vi "Teleop.vi"(10 "Match Info":T1={"Autonomous Elapsed Seconds"=0.0, "TeleOp Elapsed Seconds"=0.0, "Disabled Elapsed Seconds"=0.0, "Visited Autonomous"=FALSE, "Visited TeleOp"=FALSE, "Visited Disabled"=FALSE, "Autonomous Settings"={"Autonomous Style"=enum."Independent", "VI Refnum"=refnum}}, 11 "Call Context":T2) -> ()   [LabVIEW 2012]
doc: "This VI is called for each TeleOp packet received from the DS where the robot is not disabled. It is often used to read from the joysticks and update I/O or to update setpoints for timed control loops. It should complete and return within 20 milliseconds or it may miss DS packets."
uses:
  <vilib>/Rock Robotics/WPI/DriverStation/WPI_DriverStationDerivedRobotMode.ctl
  <vilib>/Rock Robotics/WPI/DriverStation/WPI_DriverStationMatch Info.ctl
  Desktop/Code 2013/ king-kong-2230-2013/Robot Global Data.vi
  <vilib>/Rock Robotics/WPI/RobotDrive/WPI_RobotDriveGetSetRefNum.vi
panel:
  in  "Telescopic Toghether?":bool
  in  "Cannons Toghether?":bool
  in  "Cananot Toghether?":bool
  in  "2  Cananot (Climb)":dbl(slide) scale=-1.0..1.0
  in  "2  Telescopic(Climb)":dbl(slide) scale=-1.0..1.0
  in  "2 Cannons":dbl(slide) scale=-1.0..1.0
  in  "Flipper Servos":i32(knob) scale=0.0..170.0
  in  "Feeder Servos":i32(knob) scale=0.0..160.0
  in  "Climb Telescopic Right":dbl(slide) scale=-1.0..1.0
  in  "Climb Telescopic Left":dbl(slide) scale=-1.0..1.0
  in  "Transfer":dbl(slide) scale=-1.0..1.0
  in  "Canenet Left":dbl(slide) scale=-1.0..1.0
  in  "Canenet Right":dbl(slide) scale=-1.0..1.0
  in  "Conveyer Belt":dbl(slide) scale=-1.0..1.0
  in  "zAvit":dbl(slide) scale=-1.0..1.0
  in  "First Cannon":dbl(slide) scale=-1.0..1.0
  in  "Second Cannon":dbl(slide) scale=-1.0..1.0
  in  "Y axis value":dbl(slide) scale=-1.0..1.0
  in  "X axis value":dbl(slide) scale=-1.0..1.0
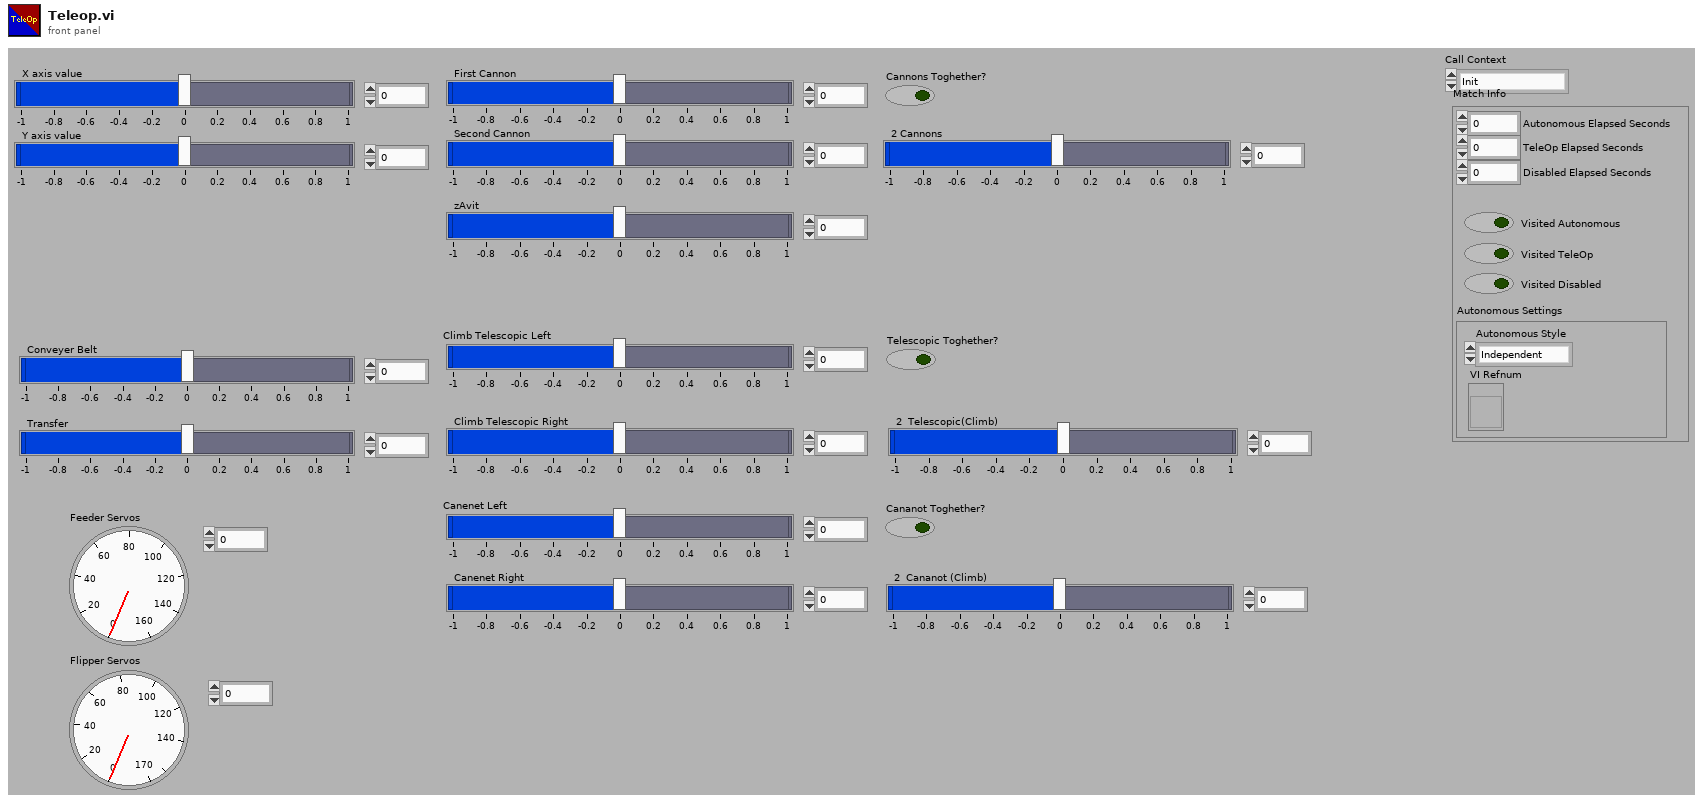
[diagram p1: front panel]
types:
  T1 = typedef "WPI_DriverStationMatch Info.ctl" = cluster{"Autonomous Elapsed Seconds":dbl, "TeleOp Elapsed Seconds":dbl, "Disabled Elapsed Seconds":dbl, "Visited Autonomous":bool, "Visited TeleOp":bool, "Visited Disabled":bool, "Autonomous Settings":cluster{"Autonomous Style":enum16{"Iterative", "Independent"}, "VI Refnum":refnum<vi>}}
  T2 = typedef "WPI_DriverStationDerivedRobotMode.ctl" = enum16{"Init", "Execute", "Stop"}
  T3 = typedef "WPI_MotorControlDeviceRef.ctl" = cluster{"DeviceStatus":errorcluster, "Type":enum16{"PWM", "CAN"}, "PWM":cluster{"Digital Module":T4, "PWM Channel":T5, "DeadBand":T6}, "CAN":cluster{"Device Number":u8, "Control Mode":T7, "Semaphore":T8, "Max Vout":dbl}, "Invert":bool, "TransformRef":T9, "InvTransformRef":T9}
  T4 = typedef "FPGA_TypedefDigitalModule.ctl" = enum16{"Digital Module 1", "Digital Module 2"}
  T5 = typedef "FPGA_DIOPWMChannel.ctl" = enum8{"PWM 1", "PWM 2", "PWM 3", "PWM 4", "PWM 5", "PWM 6", "PWM 7", "PWM 8", "PWM 9", "PWM 10", "Invalid"}
  T6 = typedef "WPI_PWMDeadband.ctl" = cluster{"Name":string, "maxPositivePwm":i32, "minPositivePwm":i32, "centerPwm":i32, "maxNegativePwm":i32, "minNegativePwm":i32, "angularRange":u16}
  T7 = typedef "WPI_CANJaguar_ControlMode.ctl" = enum8{"Percent VBus", "Current", "Speed", "Position", "Voltage"}
  T8 = typedef "Semaphore RefNum" = refnum<k1>
  T9 = typedef "WPI_PWMTransform_ConPane.ctl" = refnum<vi>
  T10 = typedef "WPI_ServoDeviceRef.ctl" = cluster{"DeviceStatus":errorcluster, "Digital Module":T4, "PWM Channel":T5, "DeadBand":T6}
  T11 = typedef "WPI_RobotDriveDevRef.ctl" = cluster{"DevStatus":errorcluster, "Motors[]":T3[], "Square Inputs":bool, "Max Output":dbl, "Isochronous":bool}
  T12 = typedef "WPI_RelayDevRef.ctl" = cluster{"DevStatus":errorcluster, "Relay Channel":T13, "Digital Module":T4, "Relay Direction":T14}
  T13 = typedef "FPGA_DIORelayChannel.ctl" = enum8{"Relay 1", "Relay 2", "Relay 3", "Relay 4", "Relay 5", "Relay 6", "Relay 7", "Relay 8", "Invalid"}
  T14 = typedef "WPI_RelayDirection.ctl" = enum16{"Both directions", "Forward only", "Reverse only"}
  T15 = typedef "WPI_RelayValue.ctl" = enum16{"Off", "On", "Forward", "Reverse"}
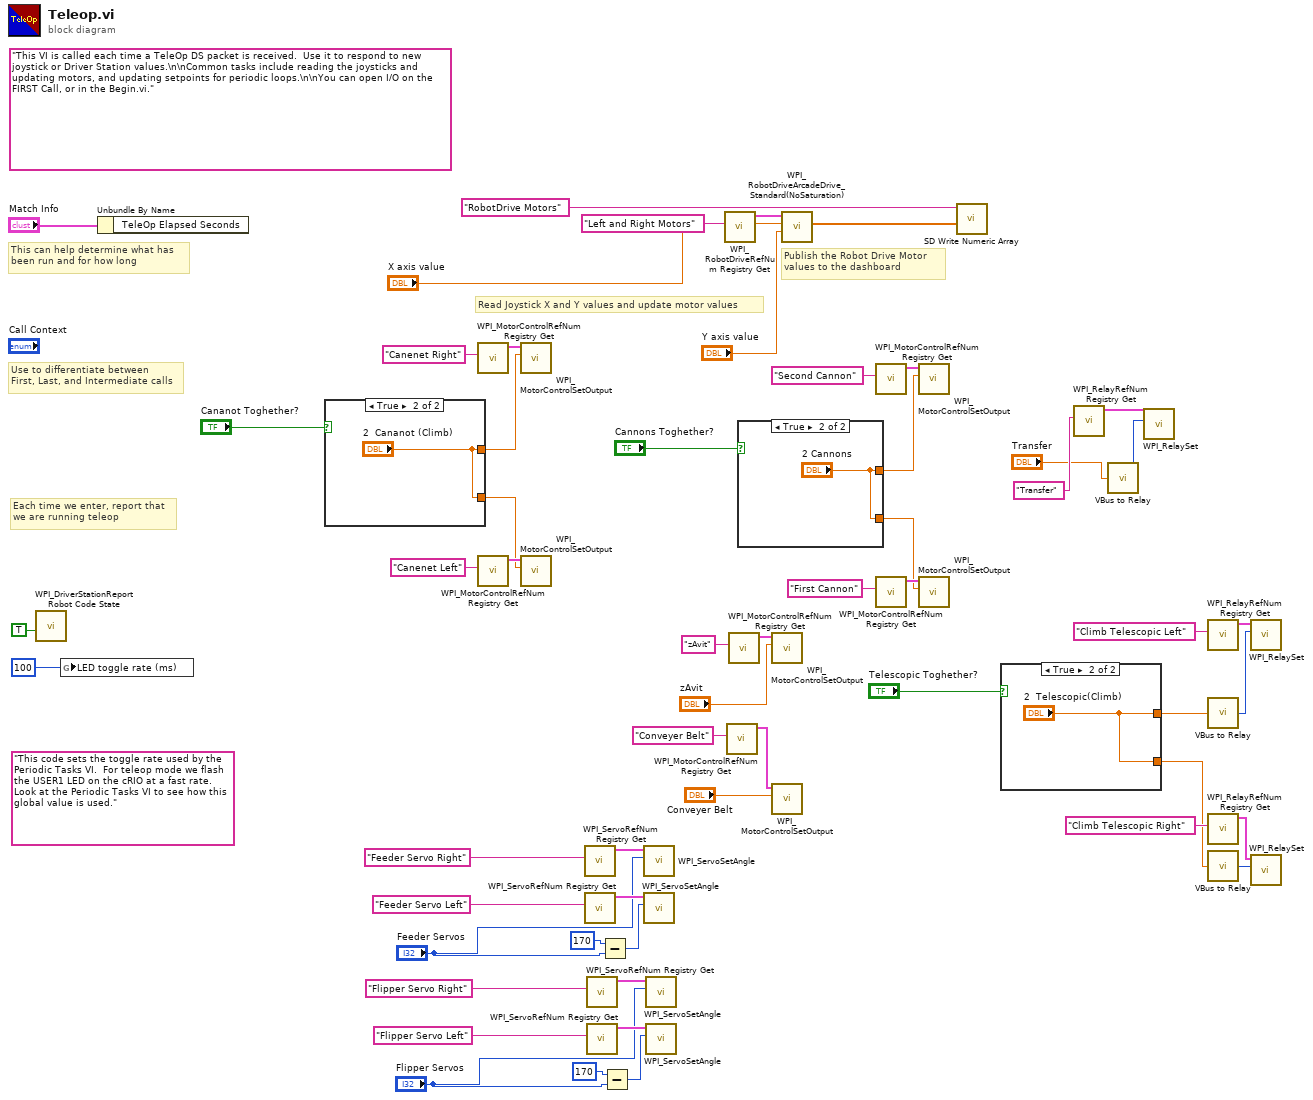
[diagram p0: block diagram]
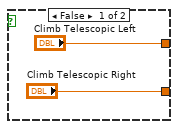
[diagram p2: hidden frame]
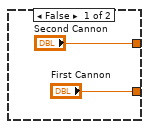
[diagram p3: hidden frame]
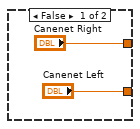
[diagram p4: hidden frame]
diagram:
  (unwired) "This code sets the toggle rate used by the Periodic Tasks VI.  For teleop mode we flash the USER1 LED on the cRIO at a fast rate.  Look at the Periodic Tasks VI to see how this global value is used."
  (unwired) "This VI is called each time a TeleOp DS packet is received.  Use it to respond to new joystick or Driver Station values.\n\nCommon tasks include reading the joysticks and updating motors, and updating setpoints for periodic loops.\n\nYou can open I/O on the FIRST Call, or in the Begin.vi."
  # "Publish the Robot Drive Motor\nvalues to the dashboard"
  # "Each time we enter, report that\nwe are running teleop"
  # "Use to differentiate between\nFirst, Last, and Intermediate calls"
  # "This can help determine what has\nbeen run and for how long"
  # "Read Joystick X and Y values and update motor values"
  n1 = call <vilib>:"WPI_DriverStationReport Robot Code State.vi"("TeleOp"=TRUE ("Autonomous")) -> ()  [unwired: 10 in, 1 out]
  n2 = global write "Robot Global Data.vi" "LED toggle rate (ms)"(u32 100 ("LED ms toggle rate")) -> ()
  n3 = Unbundle By Name("Match Info") -> ()  [unwired: 1 out]
  n4 = case shown="True" "Cananot Toghether?" {
    tunnel: ["Canenet Right" "2  Cananot (Climb)"] -> w8
    tunnel: ["Canenet Left" "2  Cananot (Climb)"] -> w7
    frame False {
    }
    frame True {
    }
  }
  n5 = call <vilib>:"WPI_MotorControlRefNum Registry Get.vi"("refnum name"="Canenet Right") -> ("MotorControlDevRef"=w28:T3)  [unwired: 9 in, 1 out]
  n6 = call <vilib>:"WPI_MotorControlRefNum Registry Get.vi"("refnum name"="Canenet Left") -> ("MotorControlDevRef"=w27:T3)  [unwired: 9 in, 1 out]
  n7 = call <vilib>:"WPI_MotorControlSetOutput.vi"("Output"=w8, "MotorControlDevRef"=w28) -> ()  [unwired: 7 in, 3 out]
  n8 = call <vilib>:"WPI_MotorControlSetOutput.vi"("Output"=w7, "MotorControlDevRef"=w27) -> ()  [unwired: 7 in, 3 out]
  n9 = call <vilib>:"WPI_ServoRefNum Registry Get.vi"("refnum name"="Feeder Servo Right") -> ("ServoDeviceRef"=w46:T10)  [unwired: 9 in, 1 out]
  n10 = call <vilib>:"WPI_ServoRefNum Registry Get.vi"("refnum name"="Feeder Servo Left") -> ("ServoDeviceRef"=w47:T10)  [unwired: 9 in, 1 out]
  n11 = call <vilib>:"WPI_ServoRefNum Registry Get.vi"("refnum name"="Flipper Servo Right") -> ("ServoDeviceRef"=w44:T10)  [unwired: 9 in, 1 out]
  n12 = call <vilib>:"WPI_ServoRefNum Registry Get.vi"("refnum name"="Flipper Servo Left") -> ("ServoDeviceRef"=w45:T10)  [unwired: 9 in, 1 out]
  n13 = Subtract(x=170, y="Feeder Servos") -> (x-y=w12:i32)
  n14 = Subtract(x=170, y="Flipper Servos") -> (x-y=w10:i32)
  n15 = call <vilib>:"WPI_ServoSetAngle.vi"("Angle"="Feeder Servos", "ServoDeviceRef"=w46) -> ()  [unwired: 8 in, 2 out]
  n16 = call <vilib>:"WPI_ServoSetAngle.vi"("Angle"=w12, "ServoDeviceRef"=w47) -> ()  [unwired: 8 in, 2 out]
  n17 = call <vilib>:"WPI_ServoSetAngle.vi"("Angle"="Flipper Servos", "ServoDeviceRef"=w44) -> ()  [unwired: 8 in, 2 out]
  n18 = call <vilib>:"WPI_ServoSetAngle.vi"("Angle"=w10, "ServoDeviceRef"=w45) -> ()  [unwired: 8 in, 2 out]
  n19 = call <vilib>:"WPI_RobotDriveRefNum Registry Get.vi"("refnum name"="Left and Right Motors") -> ("RobotDriveDevRef"=w54:T11)  [unwired: 1 in, 9 out]
  n20 = call <vilib>:"WPI_MotorControlRefNum Registry Get.vi"("refnum name"="Conveyer Belt") -> ("MotorControlDevRef"=w31:T3)  [unwired: 9 in, 1 out]
  n21 = call <vilib>:"WPI_MotorControlRefNum Registry Get.vi"("refnum name"="zAvit") -> ("MotorControlDevRef"=w35:T3)  [unwired: 9 in, 1 out]
  n22 = case shown="True" "Cannons Toghether?" {
    tunnel: ["First Cannon" "2 Cannons"] -> w5
    tunnel: ["Second Cannon" "2 Cannons"] -> w4
    frame False {
    }
    frame True {
    }
  }
  n23 = call <vilib>:"WPI_MotorControlSetOutput.vi"("Output"="zAvit", "MotorControlDevRef"=w35) -> ()  [unwired: 7 in, 3 out]
  n24 = call <vilib>:"WPI_MotorControlSetOutput.vi"("Output"="Conveyer Belt", "MotorControlDevRef"=w31) -> ()  [unwired: 7 in, 3 out]
  n25 = call <vilib>:"WPI_RobotDriveArcadeDrive_Standard(NoSaturation).vi"("Y axis value"="Y axis value", "X axis value"="X axis value", "RobotDriveDevRef"=w54) -> ("Motor Values"=w50:dbl[])  [unwired: 1 in, 7 out]
  n26 = call <vilib>:"WPI_MotorControlRefNum Registry Get.vi"("refnum name"="Second Cannon") -> ("MotorControlDevRef"=w36:T3)  [unwired: 9 in, 1 out]
  n27 = call <vilib>:"WPI_MotorControlRefNum Registry Get.vi"("refnum name"="First Cannon") -> ("MotorControlDevRef"=w39:T3)  [unwired: 9 in, 1 out]
  n28 = call <vilib>:"WPI_MotorControlSetOutput.vi"("Output"=w4, "MotorControlDevRef"=w36) -> ()  [unwired: 7 in, 3 out]
  n29 = call <vilib>:"WPI_MotorControlSetOutput.vi"("Output"=w5, "MotorControlDevRef"=w39) -> ()  [unwired: 7 in, 3 out]
  n30 = call <vilib>:"SD Write Numeric Array.vi"("Numeric Array"=w50, "Name"="RobotDrive Motors") -> ()  [unwired: 8 in, 2 out]
  n31 = case shown="True" "Telescopic Toghether?" {
    tunnel: ["Climb Telescopic Left" "2  Telescopic(Climb)"] -> w2
    tunnel: ["Climb Telescopic Right" "2  Telescopic(Climb)"] -> w1
    frame False {
    }
    frame True {
    }
  }
  n32 = call <vilib>:"WPI_RelayRefNum Registry Get.vi"("refnum name"="Transfer") -> ("RelayDevRef"=w25:T12)  [unwired: 9 in, 1 out]
  n33 = call "VBus to Relay.vi"("Motor VBus"="Transfer") -> ("RelayValue"=w22:T15)  [unwired: 3 in]
  n34 = call <vilib>:"WPI_RelaySet.vi"("RelayValue"=w22, "RelayDevRef"=w25) -> ()  [unwired: 8 in, 2 out]
  n35 = call <vilib>:"WPI_RelayRefNum Registry Get.vi"("refnum name"="Climb Telescopic Left") -> ("RelayDevRef"=w20:T12)  [unwired: 9 in, 1 out]
  n36 = call "VBus to Relay.vi"("Motor VBus"=w2) -> ("RelayValue"=w21:T15)  [unwired: 3 in]
  n37 = call <vilib>:"WPI_RelayRefNum Registry Get.vi"("refnum name"="Climb Telescopic Right") -> ("RelayDevRef"=w19:T12)  [unwired: 9 in, 1 out]
  n38 = call "VBus to Relay.vi"("Motor VBus"=w1) -> ("RelayValue"=w18:T15)  [unwired: 3 in]
  n39 = call <vilib>:"WPI_RelaySet.vi"("RelayValue"=w21, "RelayDevRef"=w20) -> ()  [unwired: 8 in, 2 out]
  n40 = call <vilib>:"WPI_RelaySet.vi"("RelayValue"=w18, "RelayDevRef"=w19) -> ()  [unwired: 8 in, 2 out]
